vi "LWXPS_ControllerMotionKernelTimeLoadGet.vi"(1 "XPS Reference IN":refnum<k24>, 4 "LabVIEW error IN":errorcluster) -> (12 "XPS Reference OUT":refnum<k24>, 13 "LabVIEW error OUT":errorcluster, 14 "Returned error code":i32, 15 "CPU Total Load Ratio":dbl, 16 "CPU Corrector Load Ratio":dbl, 17 "CPU Profiler Load Ratio":dbl, 18 "CPU Servitudes Load Ratio":dbl, 19 "XPS Error String":string)   [LabVIEW 2014]
uses:
  D:/XPSQ8_LabView_Library/Development/Source/Dll/Newport.XPS.CommandInterface.dll
  Dll/Newport.XPS.CommandInterface.dll
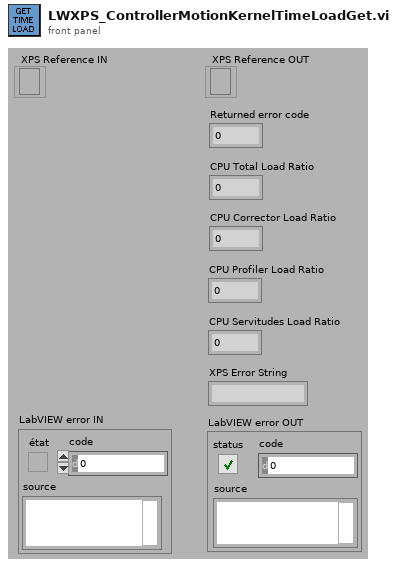
[diagram p1: front panel]
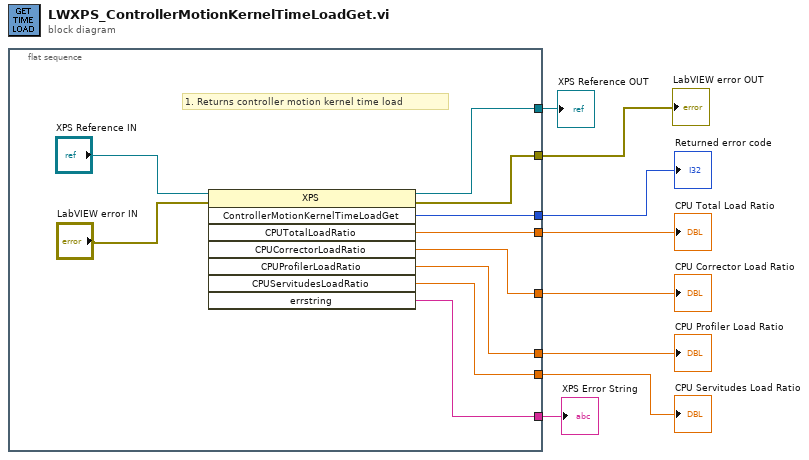
[diagram p0: block diagram]
diagram:
  n1 = flat-sequence {
    tunnel: [w16] -> w8
    tunnel: [w18] -> w7
    tunnel: [w17] -> w5
    tunnel: [w13] -> w6
    tunnel: [w12] -> w4
    tunnel: [w11] -> w3
    tunnel: [w10] -> w2
    tunnel: [w9] -> w1
    frame #0 {
      # "1. Returns controller motion kernel time load"
      n2 = invoke class="XPS" method="ControllerMotionKernelTimeLoadGet"(reference="XPS Reference IN", error in="LabVIEW error IN") -> (reference out=w16:refnum<k24>, error out=w18:errorcluster, "ControllerMotionKernelTimeLoadGet"=w13:i32, "CPUTotalLoadRatio"=w17:dbl, "CPUCorrectorLoadRatio"=w12:dbl, "CPUProfilerLoadRatio"=w11:dbl, "CPUServitudesLoadRatio"=w10:dbl, "errstring"=w9:string)  [unwired: 6 in]
    }
  }
  "XPS Reference OUT" <- w8
  "LabVIEW error OUT" <- w7
  "Returned error code" <- w6
  "CPU Total Load Ratio" <- w5
  "CPU Corrector Load Ratio" <- w4
  "CPU Profiler Load Ratio" <- w3
  "CPU Servitudes Load Ratio" <- w2
  "XPS Error String" <- w1
